vi "rs3 create context2.vi"(8 "error in (no error)":errorcluster, 11 "version":i32=20000) -> (0 "error out":errorcluster, 3 "context":u32)   [LabVIEW 2023]
doc: "This has to be the first call to initialize libRealSense. \nThe input is the Version Check for the libRealSense, and the output is the Context that needs to be passed to Device Count and Get Device, etc."
panel:
  # "RS3 Create Context2"
  # "(C) Intel Corp.,  AGJ"
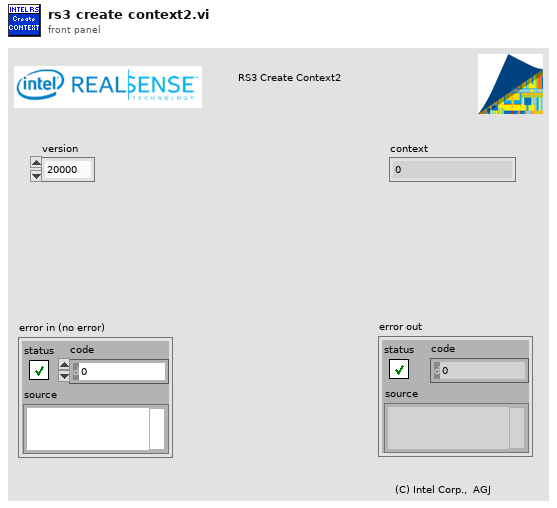
[diagram p1: front panel]
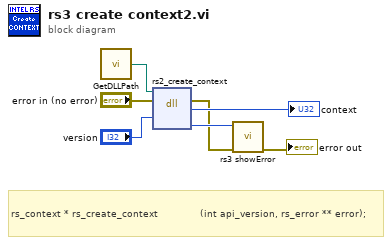
[diagram p0: block diagram]
diagram:
  # "rs_context * rs_create_context              (int api_version, rs_error ** error);"
  n1 = call "GetDLLPath.vi"() -> ("DLL Path"=w1:path)
  n2 = dll-call lib="C:/STEAMSyndicate/RealSenseWrappers/VI Wrappers (add ons) Public/RealSense/realsense2.dll" fn="rs2_create_context"(path in=w1, error in="error in (no error)", "api_version"="version") -> (error out=w2:errorcluster, "context"=→"context":u64, "error"=w3:u64)  [unwired: 3 in, 1 out]
  n3 = call "rs3 showError.vi"("error in (no error)"=w2, "error"=w3) -> ("error out"=→"error out":errorcluster)  [unwired: 5 in, 4 out]
